vi "Integer Check Squares.vi"(11 "Sudoku Int":u8[][](array[numeric])) -> (3 "Is Ok":bool)   [LabVIEW 2015, in "Sudoku Library.lvlib"]
doc: "Created IvanLis by LabVIEW Portal\nProfile: http://labviewportal.org/memberlist.php?mode=viewprofile&u=987\neMail: IvanLisanov@gMail.com\nTelegram: https://t.me/IvanLis"
uses:
  Sudoku Library.lvlib
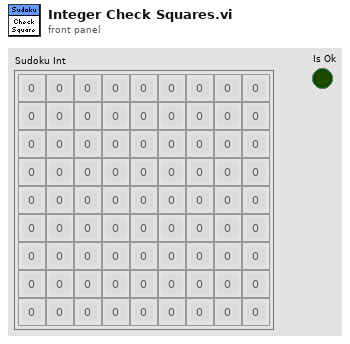
[diagram p1: front panel]
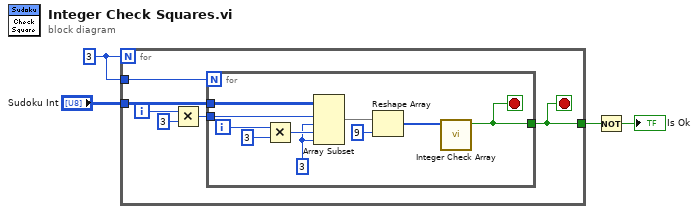
[diagram p0: block diagram]
diagram:
  w1 = 3
  n1 = for {
    N: w1 -> [_]
    tunnel: "Sudoku Int" -> [w10]
    tunnel: [w9] -> w3
    tunnel: w1 -> [w8]
    i -> [w7]
    stop <- w9 stop-if-true
    n2 = Multiply(x=w7, y=3) -> (x*y=w5:i32)
    n3 = for {
      N: w8 -> [_]
      tunnel: w10 -> [w20]
      tunnel: [w11] -> w9
      tunnel: w5 -> [w19]
      i -> [w16]
      stop <- w11 stop-if-true
      w15 = 3 ("y")
      n4 = Multiply(x=w16, y=3) -> (x*y=w17:i32)
      n5 = Array Subset(array=w20, index (row)=w19, length (row)=w15, index (col)=w17, length (col)=w15) -> (w14:u8[][])
      n6 = Reshape Array(w14, 9 ("dimension size")) -> (w12:u8[])
      n7 = call "Integer Check Array.vi"("Array"=w12) -> ("Error"=w11:bool)  [unwired: 10 in]
    }
  }
  n8 = Not(x=w3) -> (.not. x?=→"Is Ok":bool)
